vi "Filter Hysteresis Results.vi"(8 "error in (no error)":errorcluster, 10 "SensorID":i32, 11 "Hysteresis Results":T1[](array[typedef])) -> (0 "error out":errorcluster, 3 "Filtered Hysteresis":T1[](array[typedef]))   [LabVIEW 2026, in "Analysis.lvlib"]
uses:
  Analysis.lvlib
  Hysteresis Result.ctl
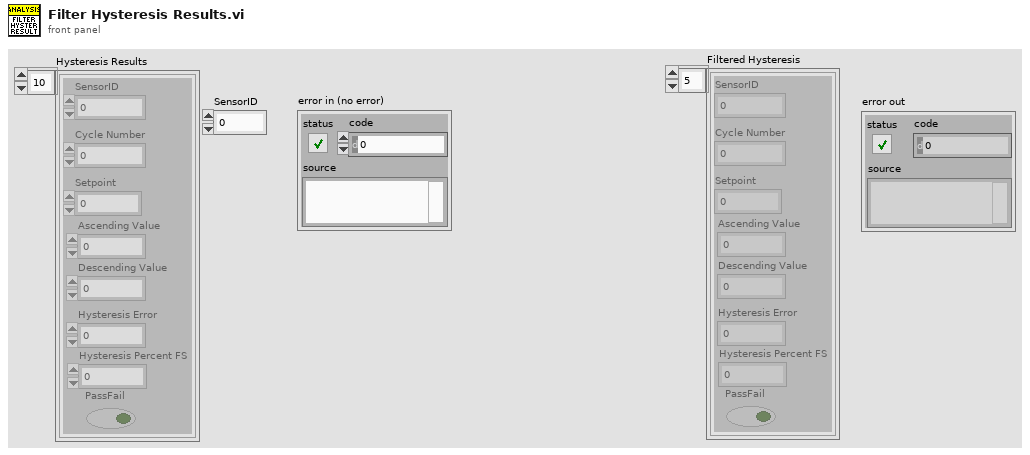
[diagram p1: front panel]
types:
  T1 = typedef "Analysis.lvlib/Hysteresis Result.ctl" = cluster{"Setpoint":dbl, "Ascending Value":dbl, "Cycle Number":i32, "SensorID":i32, "Descending Value":dbl, "Hysteresis Error":dbl, "Hysteresis Percent FS":dbl, "PassFail":bool}
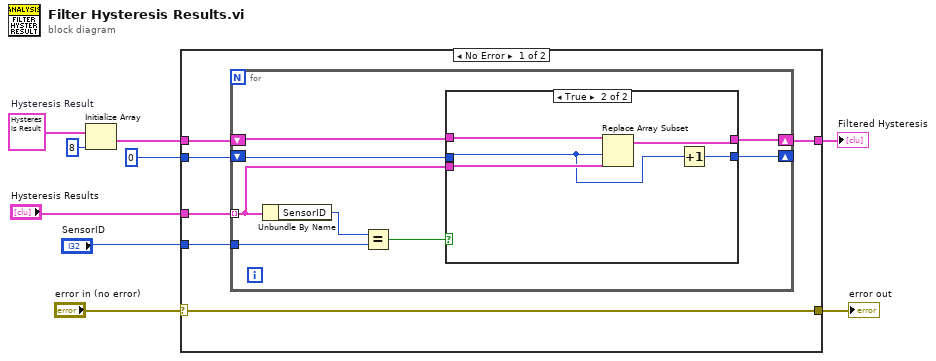
[diagram p0: block diagram]
diagram:
  w6 = T1 {"Setpoint"=-0.000162682555527026, "Ascending Value"=4.94667402746659, "Cycle Number"=0, "SensorID"=18, "Descending Value"=0.0, "Hysteresis Error"=4.94667402746659, "Hysteresis Percent FS"=0.0, "PassFail"=FALSE}  # Hysteresis Result
  n1 = Initialize Array(w6, 8 ("dimension size")) -> (w5:T1[])
  n2 = case shown="No Error" "error in (no error)" {
    selector: "error in (no error)" -> [w10 w32]
    tunnel: "SensorID" -> [w15 _]
    tunnel: "Hysteresis Results" -> [w14 _]
    tunnel: [w13 w31] -> w7
    tunnel: w5 -> [w12 w31]
    tunnel: 0 -> [w11 _]
    tunnel: [w10 w32] -> w1
    frame No Error {
      n3 = for {
        tunnel: w14 -> [w20] mode=indexing
        tunnel: w15 -> [w22]
        shift-right: [w18] -> w13
        shift-left: w12 -> [w19]
        shift-right: [w16] -> _
        shift-left: w11 -> [w17]
        n4 = Unbundle By Name(w20) -> ("SensorID"=w23:i32)
        n5 = Equal?(x=w23, y=w22) -> (x = y?=w21:bool)
        n6 = case shown="True" w21 {
          tunnel: w20 -> [_ w28]
          tunnel: w19 -> [w25 w30]
          tunnel: [w25 w29] -> w18
          tunnel: w17 -> [w24 w27]
          tunnel: [w24 w26] -> w16
          frame False {
          }
          frame True {
            n7 = Replace Array Subset(array=w30, new element=w28, index=w27) -> (w29:T1[])
            n8 = Increment(x=w27) -> (x+1=w26:i32)
          }
        }
      }
    }
    frame Error {
    }
  }
  "Filtered Hysteresis" <- w7
  "error out" <- w1
